vi "ESP32 BLE Client - Bluegiga.vi"() -> ()   [LabVIEW 2016]
uses:
  Typedef/BLE - State.ctl
  <vilib>/BLE/type_def/connection_status_bundle.ctl
  <vilib>/BLE/type_def/address_type.ctl
  Typedef/BLE - ADC Resolution.ctl
panel:
  in  "Exit":bool
  in  "Tab":T1(tab)
  in  "Discover":bool
  in  "USB BLE Dongle port":refnum<visa-resource-name>
  out "Dongle Status":bool
  in  "Connect dongle":bool
  out "BLED112 Dongle Info":string
  in  "MAC Address":string="24:0A:C4:04:1C:4E"
  in  "Address type":enum8{"Public", "Random"}(ring)
  in  "Connect BLE":bool
  out "BLE Status":bool
  out "Devices":i32(listbox)=-1
  in  "Min interval":u16=20 caption="Connection interval (min)" min=10 max=4000 step=1 format="%.0fms"
  in  "Max interval":u16=50 caption="Connection interval (max)" min=10 max=4000 step=1 format="%.0fms"
  in  "Latency":u16 max=500 step=1
  in  "Timeout":u16=1000 format="%.0fms"
  out "Gatt server table":i32(listbox)=-1
  in  "Single read":bool
  in  "Stream data":bool
  out "Data chart":T2(graph)
  in  "Acq interval":u32=50 min=50 max=100 step=5 format="%.0fms"
  out "Read Value":u32 caption="Read Value (Max 4 Bytes)" format="%08x"
  out "Cycle time":u32 format="%.0fms"
  in  "Clear Plot":bool
  in  "Handle":u16=42 format="%04x"
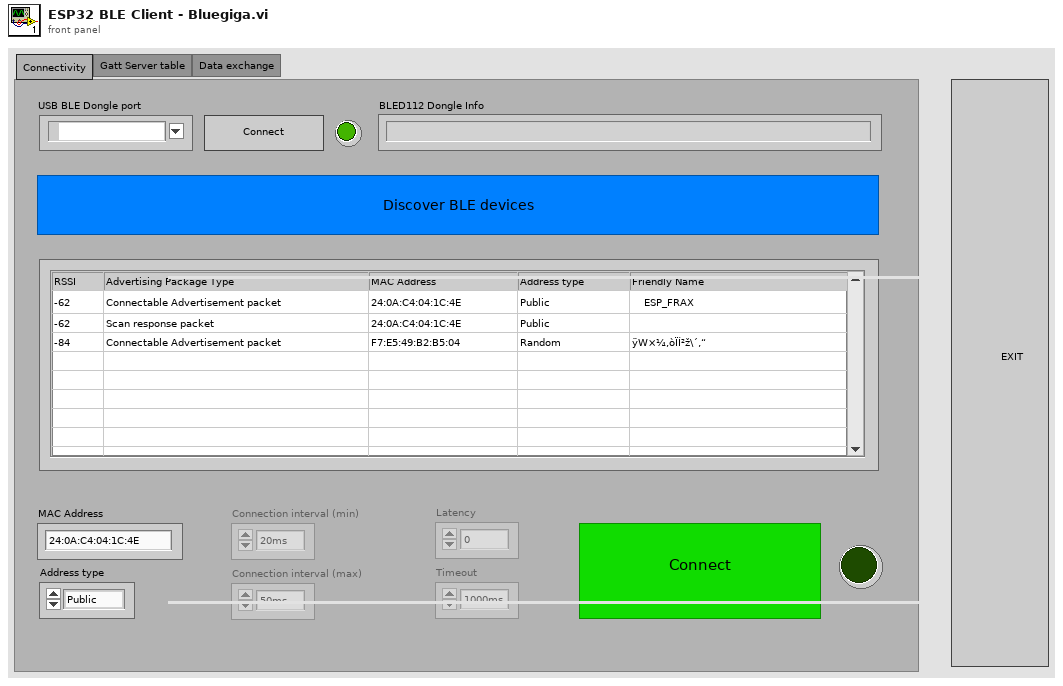
[diagram p1: front panel]
types:
  T1 = enum32{"Connectivity", "Gatt Server table", "Data exchange"}
  T2 = cluster{"Data value[0]":sgl, "Data value[1]":sgl}
  T3 = typedef "connection_status_bundle.ctl" = cluster{"MAC Address":string, "cnx handle":u8, "cnx flags":u8, "Address Type":T4, "Connection Interval (ms)":u16, "Timeout(ms)":u16, "Latency":u16, "bonding handle":u8}
  T4 = typedef "address_type.ctl" = u8
  T5 = cluster{"Connection Status":T3, "MAC Address":string, "Handle table":string[][], "Is Connected":bool}
  T6 = typedef "BLE - State.ctl" = enum16{"Connect Dongle", "Discover BLE", "Connect BLE", "Disconnect BLE", "Discover Services", "Single read", "Stream Data", "Stop Data", "Exit"}
  T7 = cluster{"Data value[0]":sgl, "Data value[1]":sgl}[]
  T8 = typedef "BLE - ADC Resolution.ctl" = enum16{"9bit", "10bit", "11bit", "12bit"}
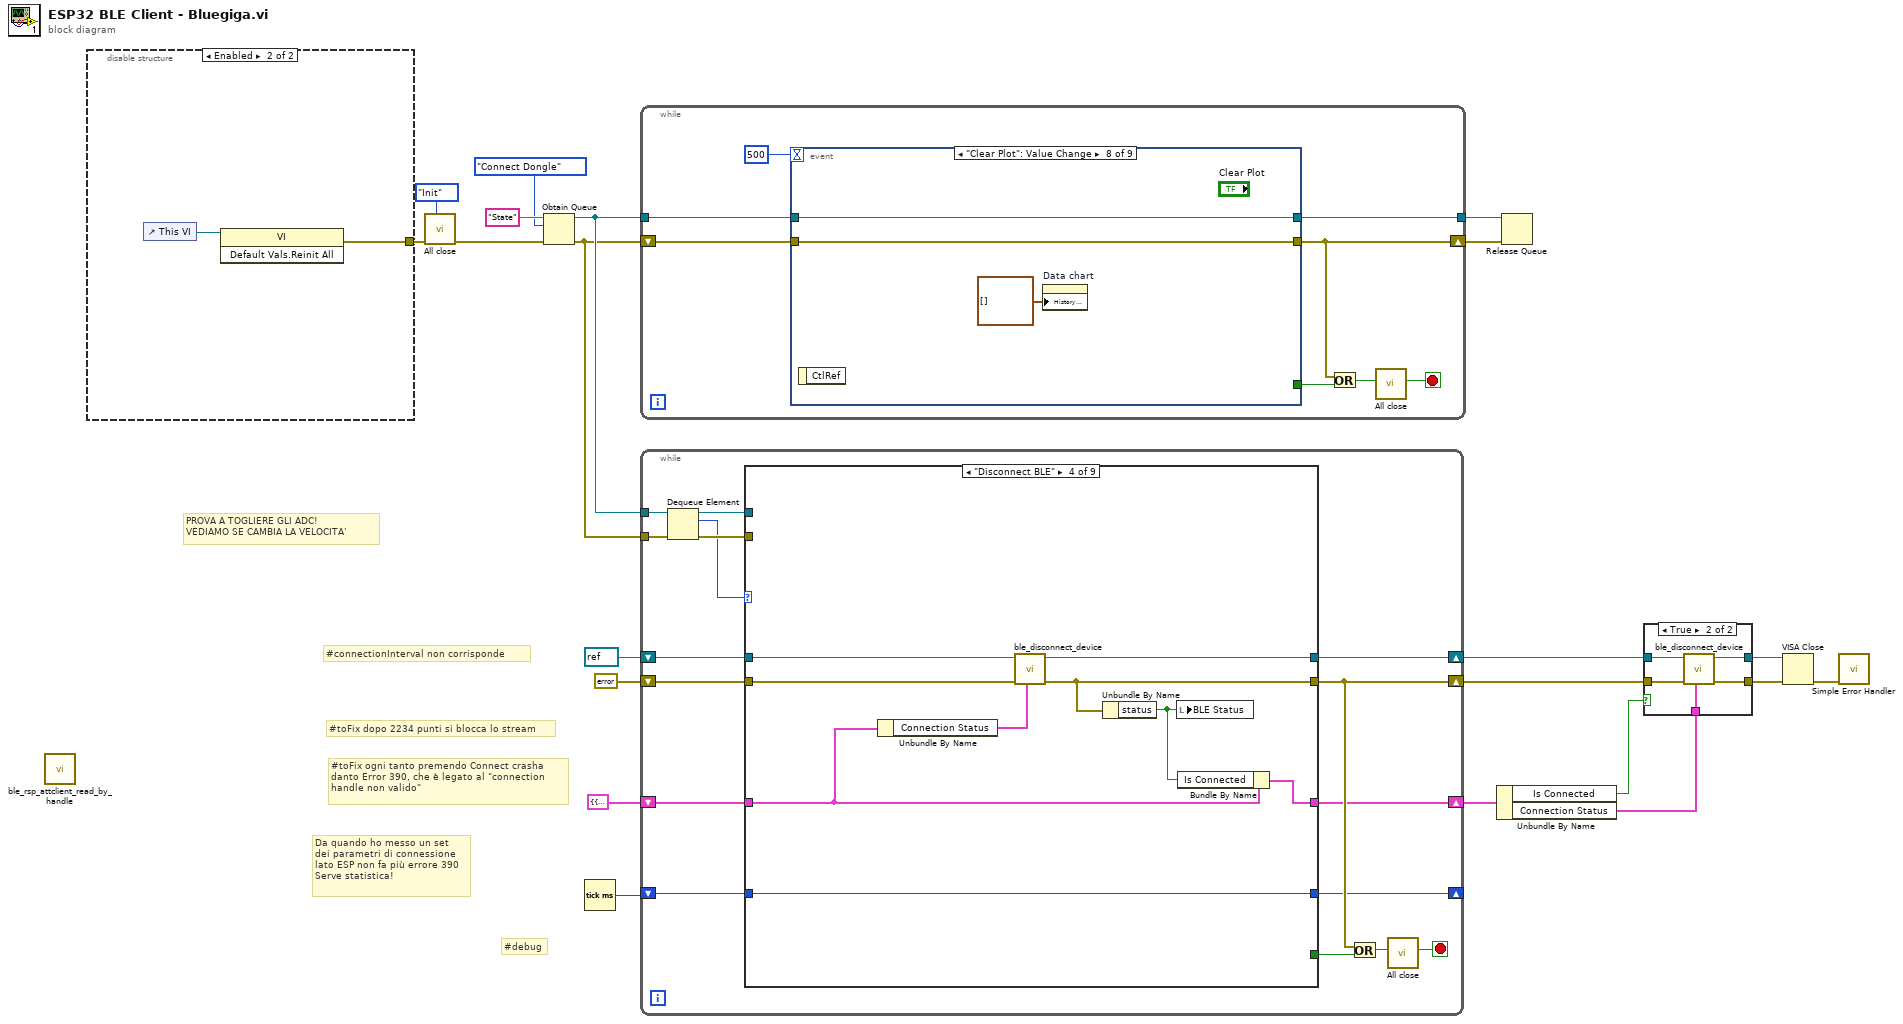
[diagram p0: block diagram]
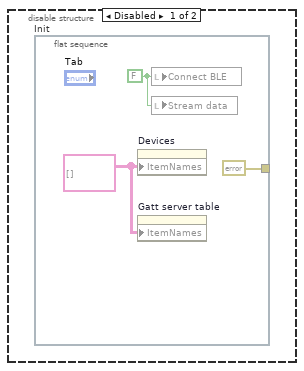
[diagram p2: hidden frame]
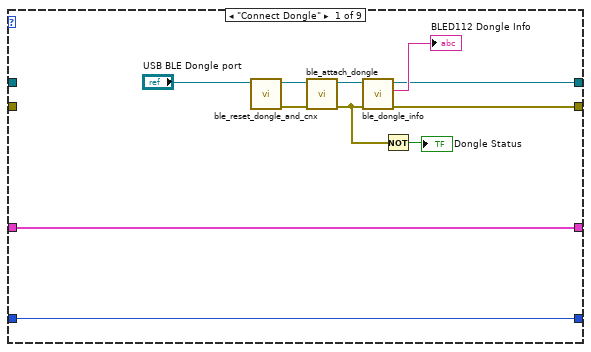
[diagram p4: hidden frame]
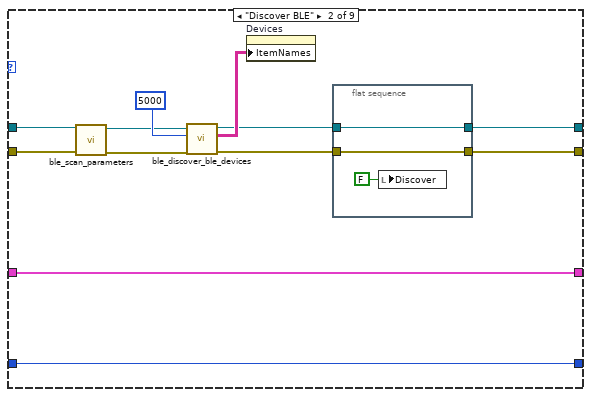
[diagram p5: hidden frame]
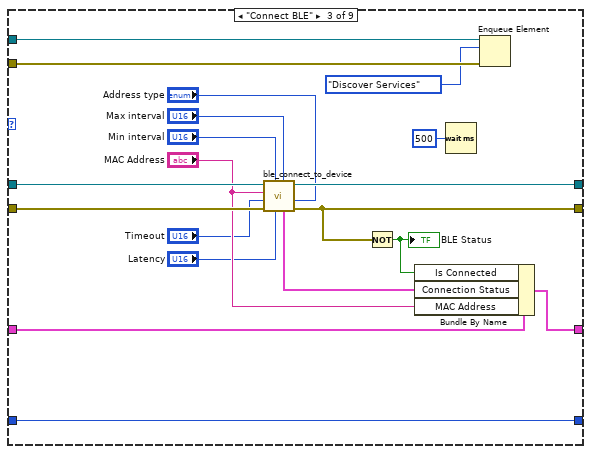
[diagram p6: hidden frame]
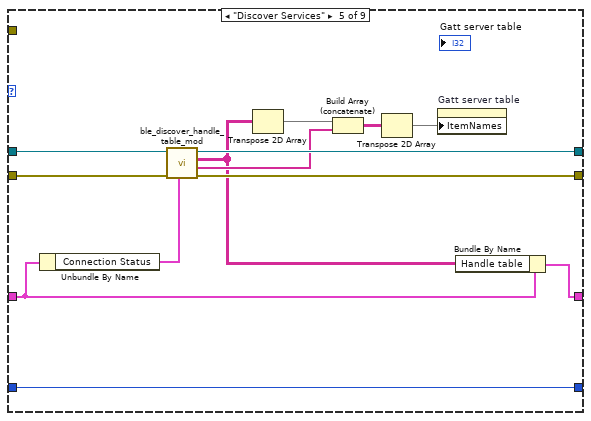
[diagram p7: hidden frame]
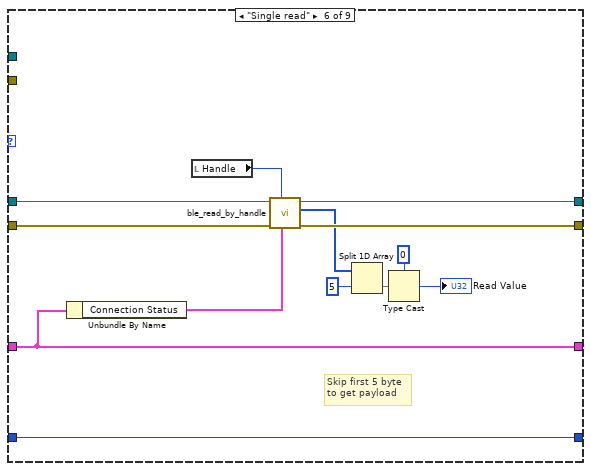
[diagram p8: hidden frame]
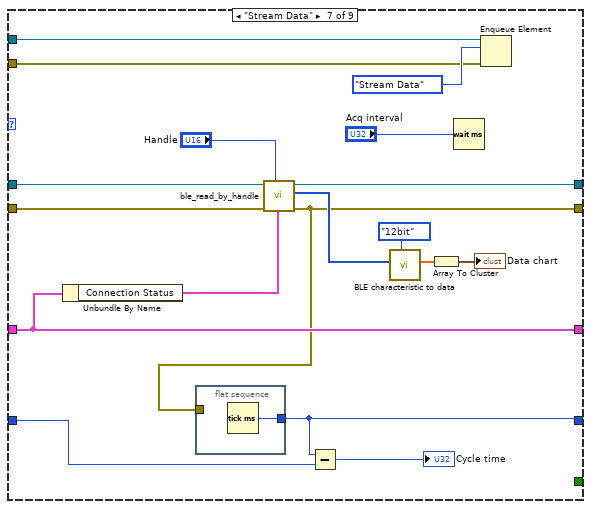
[diagram p9: hidden frame]
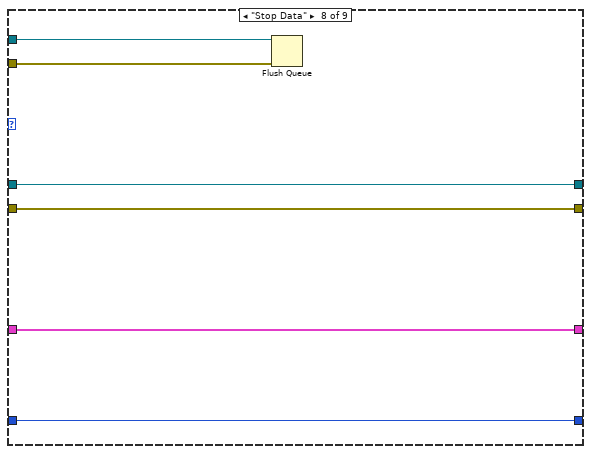
[diagram p10: hidden frame]
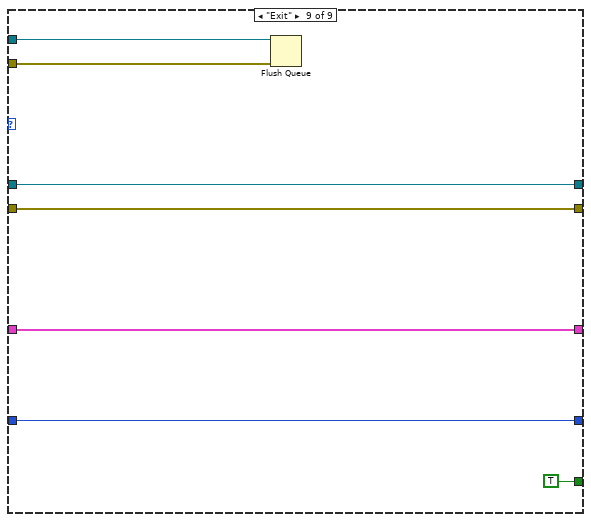
[diagram p11: hidden frame]
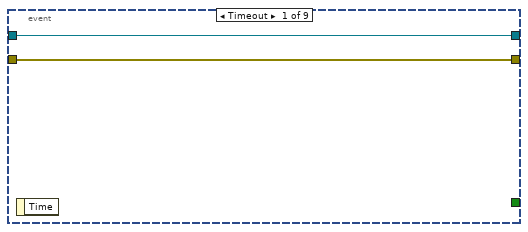
[diagram p12: hidden frame]
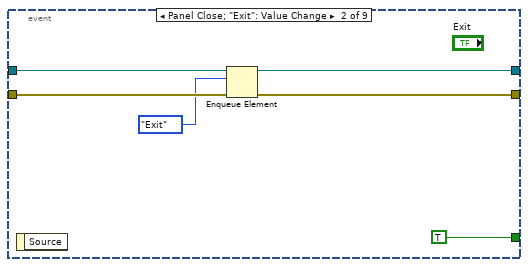
[diagram p13: hidden frame]
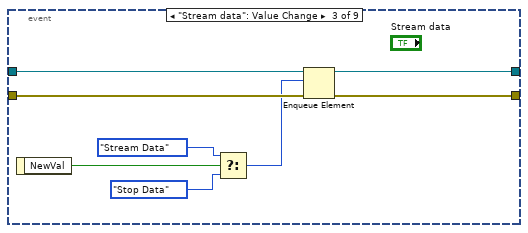
[diagram p14: hidden frame]
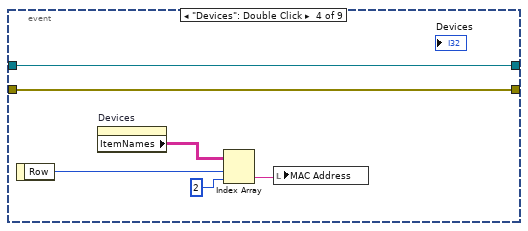
[diagram p15: hidden frame]
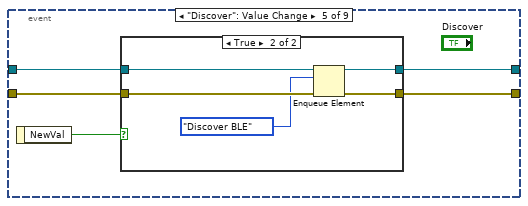
[diagram p16: hidden frame]
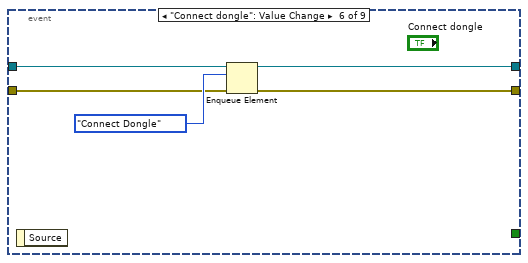
[diagram p18: hidden frame]
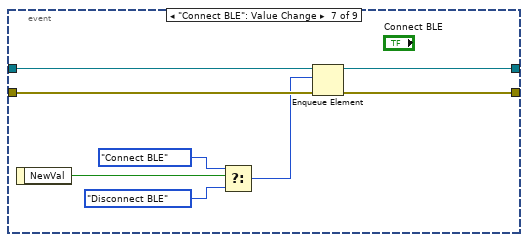
[diagram p19: hidden frame]
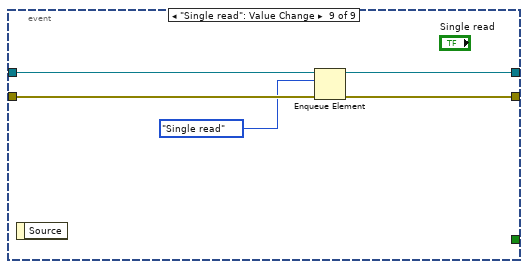
[diagram p20: hidden frame]
diagram:
  # "PROVA A TOGLIERE GLI ADC!\nVEDIAMO SE CAMBIA LA VELOCITA'"
  # "#debug"
  # "Da quando ho messo un set\ndei parametri di connessione\nlato ESP non fa più errore 390\nServe statistica!"
  # "#toFix ogni tanto premendo Connect crasha\ndanto Error 390, che è legato al \"connection\nhandle non valido\""
  # "#toFix dopo 2234 punti si blocca lo stream"
  # "#connectionInterval non corrisponde"
  n1 = call <vilib>:"ble_rsp_attclient_read_by_handle.vi"() -> ()  [unwired: 8 in, 4 out]
  n2 = disable-structure shown="Enabled" {
    disable-tunnel: [_ w25] -> w1
    frame Disabled {
      n3 = flat-sequence "Init" {
        tunnel: [errorcluster {"status"=FALSE, "code"=0, "source"=""} ("Error In")] -> _
        frame #0 {
          w22 = FALSE ("Connect BLE")
          w23 = string[][] [] ("Item Names")
          n4 = property on="Devices" class="MCListbox (strict)"("ItemNames"=w23) -> ()  [unwired: 2 in, 2 out]
          n5 = property on="Gatt server table" class="MCListbox (strict)"("ItemNames"=w23) -> ()  [unwired: 2 in, 2 out]
          n6 = local write "Connect BLE"(w22) -> ()
          n7 = local write "Stream data"(w22) -> ()
        }
      }
    }
    frame Enabled {
      n8 = control-ref of="This VI"() -> (w26:refnum<vi>)
      n9 = invoke class="VI" method="Default Vals.Reinit All"(reference=w26) -> (error out=w25:errorcluster)  [unwired: 2 in, 2 out]
    }
  }
  n10 = call "All close.vi"("Operation (Check)"=enum16{"Init", "Check"}."Init", "Error In"=w1) -> ("Error Out"=w12:errorcluster)  [unwired: 8 in, 1 out]
  n11 = Obtain Queue(name (unnamed)="State", element data type=BLE_-_State."Connect Dongle", error in (no error)=w12) -> (queue out=w18:refnum<queue>, error out=w17:errorcluster)  [unwired: 2 in, 1 out]
  n12 = Tick Count (ms)() -> (millisecond timer value=w2:u32)
  n13 = while {
    tunnel: w18 -> [w32]
    shift-right: [w29] -> w19
    shift-left: w17 -> [w33]
    tunnel: [w31] -> w20
    stop <- w27 stop-if-true
    n14 = event shown="[7] \"Clear Plot\": Value Change" {
      selector: _ -> [_ _ _ _ _ _ _ _ _]
      dyn-events: _ -> [_ _ _ _ _ _ _ _ _]
      timeout: 500 -> [_ _ _ _ _ _ _ _ _]
      tunnel: w33 -> [w35 w42 w49 w52 w60 w71 w80 w83 w88]
      tunnel: w32 -> [w36 w39 w50 w51 w61 w72 w81 w84 w89]
      tunnel: [w36 w38 w48 w51 w59 w69 w78 w84 w86] -> w31
      tunnel: [w35 w40 w47 w52 w58 w70 w79 w83 w87] -> w29
      tunnel: [_ TRUE _ _ _ _ _ _ _] -> w30
      event Timeout {
        n15 = event-data() -> ()  [unwired: 1 in, 1 out]
      }
      event Panel Close; "Exit": Value Change {
        n16 = event-data() -> ()  [unwired: 1 in, 1 out]
        n17 = Enqueue Element(queue=w39, element=BLE_-_State."Exit", error in (no error)=w42) -> (queue out=w38:refnum<queue>, error out=w40:errorcluster)  [unwired: 1 in, 1 out]
      }
      event "Stream data": Value Change {
        n18 = event-data() -> ("NewVal"=w46:bool)  [unwired: 1 in]
        n19 = Select(t=BLE_-_State."Stream Data" ("element"), s=w46, f=BLE_-_State."Stop Data") -> (s? t:f=w45:T6)
        n20 = Enqueue Element(queue=w50, element=w45, error in (no error)=w49) -> (queue out=w48:refnum<queue>, error out=w47:errorcluster)  [unwired: 1 in, 1 out]
      }
      event "Devices": Double Click {
        n21 = event-data() -> ("Row"=w55:i32)  [unwired: 1 in]
        n22 = property on="Devices" class="MCListbox (strict)"() -> ("ItemNames"=w54:string[][])  [unwired: 2 in, 2 out]
        n23 = Index Array(array=w54, index (row)=w55, index (col)=2 ("disabled index (col)")) -> (element=w53:string)
        n24 = local write "MAC Address"(w53) -> ()
      }
      event "Discover": Value Change {
        n25 = event-data() -> ("NewVal"=w57:bool)  [unwired: 1 in]
        n26 = case shown="True" w57 {
          tunnel: w61 -> [w63 w68]
          tunnel: w60 -> [w62 w67]
          tunnel: [w63 w66] -> w59
          tunnel: [w62 w65] -> w58
          frame False {
          }
          frame True {
            n27 = Enqueue Element(queue=w68, element=BLE_-_State."Discover BLE", error in (no error)=w67) -> (queue out=w66:refnum<queue>, error out=w65:errorcluster)  [unwired: 1 in, 1 out]
          }
        }
      }
      event "Connect dongle": Value Change {
        n28 = event-data() -> ()  [unwired: 1 in, 1 out]
        n29 = Enqueue Element(queue=w72, element=BLE_-_State."Connect Dongle", error in (no error)=w71) -> (queue out=w69:refnum<queue>, error out=w70:errorcluster)  [unwired: 1 in, 1 out]
      }
      event "Connect BLE": Value Change {
        n30 = event-data() -> ("NewVal"=w77:bool)  [unwired: 1 in]
        n31 = Select(t=BLE_-_State."Connect BLE", s=w77, f=BLE_-_State."Disconnect BLE" ("element")) -> (s? t:f=w74:T6)
        n32 = Enqueue Element(queue=w81, element=w74, error in (no error)=w80) -> (queue out=w78:refnum<queue>, error out=w79:errorcluster)  [unwired: 1 in, 1 out]
      }
      event "Clear Plot": Value Change {
        n33 = event-data() -> ()  [unwired: 1 in, 1 out]
        n34 = property on="Data chart" class="WFChart (strict)"("History Data"=T7 []) -> ()  [unwired: 2 in, 2 out]
      }
      event "Single read": Value Change {
        n35 = event-data() -> ()  [unwired: 1 in, 1 out]
        n36 = Enqueue Element(queue=w89, element=BLE_-_State."Single read" ("t"), error in (no error)=w88) -> (queue out=w86:refnum<queue>, error out=w87:errorcluster)  [unwired: 1 in, 1 out]
      }
    }
    n37 = Or(x=w29, y=w30) -> (x .or. y?=w28:bool)
    n38 = call "All close.vi"("Close? (F)"=w28) -> ("Close"=w27:bool)  [unwired: 9 in, 1 out]
  }
  n39 = while {
    tunnel: w18 -> [w105]
    tunnel: w17 -> [w104]
    shift-right: [w97] -> w8
    shift-left: errorcluster {"status"=FALSE, "code"=0, "source"=""} ("error out") -> [w98]
    shift-right: [w100] -> w9
    shift-left: refnum<visa-resource-name> refnum ("COM Bluegiga out") -> [w99]
    shift-right: [w94] -> w5
    shift-left: T5 {"Connection Status"={"MAC Address"="", "cnx handle"=0, "cnx flags"=0, "Address Type"=125, "Connection Interval (ms)"=125, "Timeout(ms)"=125, "Latency"=0, "bonding handle"=0}, "MAC Address"="", "Handle table"=[], "Is Connected"=FALSE} -> [w95]
    shift-right: [w90] -> _
    shift-left: w2 -> [w91]
    stop <- w92 stop-if-true
    n40 = Dequeue Element(queue=w105, error in (no error)=w104) -> (queue out=w102:refnum<queue>, element=w101:T6, error out=w103:errorcluster)  [unwired: 1 in, 1 out]
    n41 = case shown="\"Disconnect BLE\"" w101 {
      tunnel: w103 -> [_ _ w142 _ _ _ w202 w208 w212]
      tunnel: w102 -> [_ _ w143 _ _ _ w201 w209 w213]
      tunnel: [w111 w123 w148 w157 w169 w176 w190 w207 w217] -> w100
      tunnel: [w110 w124 w146 w155 w170 w177 w186 w206 w216] -> w97
      tunnel: w99 -> [_ w121 w150 w159 w168 w179 w192 w207 w217]
      tunnel: w98 -> [_ w120 w149 w158 w167 w178 w191 w206 w216]
      tunnel: [_ _ _ _ _ _ _ _ TRUE] -> w96
      tunnel: w95 -> [w112 w127 w145 w153 w172 w184 w200 w210 w214]
      tunnel: [w112 w127 w144 w152 w171 w184 w200 w210 w214] -> w94
      tunnel: w91 -> [w106 w117 w132 w154 w160 w185 w198 w205 w211]
      tunnel: [w106 w117 w132 w154 w160 w185 w195 w205 w211] -> w90
      frame "Connect Dongle" {
        n42 = call <vilib>:"ble_reset_dongle_and_cnx.vi"("COM Bluegiga in"="USB BLE Dongle port") -> ("error out"=w115:errorcluster, "COM Bluegiga out"=w108:refnum<visa-resource-name>)  [unwired: 9 in]
        n43 = call <vilib>:"ble_attach_dongle.vi"("error in (no error)"=w115, "COM Bluegiga in"=w108) -> ("error out"=w113:errorcluster, "COM Bluegiga out"=w107:refnum<visa-resource-name>)  [unwired: 8 in]
        n44 = call <vilib>:"ble_dongle_info.vi"("error in (no error)"=w113, "COM Bluegiga in"=w107) -> ("error out"=w110:errorcluster, "info"=→"BLED112 Dongle Info":string, "COM Bluegiga out"=w111:refnum<visa-resource-name>)  [unwired: 7 in]
        n45 = Not(x=w113) -> (.not. x?=→"Dongle Status":bool)
      }
      frame "Discover BLE" {
        n46 = call <vilib>:"ble_scan_parameters.vi"("error in (no error)"=w120, "COM Bluegiga in"=w121) -> ("error out"=w119:errorcluster, "COM Bluegiga out"=w118:refnum<visa-resource-name>)  [unwired: 7 in, 1 out]
        n47 = call <vilib>:"ble_discover_ble_devices.vi"("error in (no error)"=w119, "Scan Duration (10000ms)"=u32 5000, "COM Bluegiga in"=w118) -> ("error out"=w125:errorcluster, "Devices"=w126:string[][], "COM Bluegiga out"=w122:refnum<visa-resource-name>)  [unwired: 6 in]
        n48 = property on="Devices" class="MCListbox (strict)"("ItemNames"=w126) -> ()  [unwired: 2 in, 2 out]
        n49 = flat-sequence {
          tunnel: w125 -> [w130]
          tunnel: [w130] -> w124
          tunnel: [w129] -> w123
          tunnel: w122 -> [w129]
          frame #0 {
            n50 = local write "Discover"(FALSE ("Discover")) -> ()
          }
        }
      }
      frame "Connect BLE" {
        n51 = call <vilib>:"ble_connect_to_device.vi"("Address Type"="Address type", "Connection Interval Max (95ms)"="Max interval", "Latency(0)"="Latency", "Connection Interval Min (75ms)"="Min interval", "error in (no error)"=w149, "Timeout(1000ms)"="Timeout", "MAC Address"="MAC Address", "COM Bluegiga in"=w150) -> ("error out"=w146:errorcluster, "COM Bluegiga out"=w148:refnum<visa-resource-name>, "Connection Status"=w140:T3)  [unwired: 1 in]
        n52 = Not(x=w146) -> (.not. x?=w133:bool)
        "BLE Status" <- w133
        n53 = Bundle By Name(cluster=w145, "Is Connected"=w133, "Connection Status"=w140, "MAC Address"="MAC Address") -> (w144:T5)
        n54 = Wait (ms)(milliseconds to wait=u32 500) -> ()  [unwired: 1 out]
        n55 = Enqueue Element(queue=w143, element=BLE_-_State."Discover Services", error in (no error)=w142) -> ()  [unwired: 1 in, 3 out]
      }
      frame "Disconnect BLE" {
        n56 = Unbundle By Name(w153) -> ("Connection Status"=w156:T3)
        n57 = call <vilib>:"ble_disconnect_device.vi"("Connection Status"=w156, "error in (no error)"=w158, "COM Bluegiga in"=w159) -> ("error out"=w155:errorcluster, "COM Bluegiga out"=w157:refnum<visa-resource-name>)  [unwired: 7 in]
        n58 = Unbundle By Name(w155) -> ("status"=w151:bool)
        n59 = local write "BLE Status"(w151) -> ()
        n60 = Bundle By Name(cluster=w153, "Is Connected"=w151) -> (w152:T5)
      }
      frame "Discover Services" {
        n61 = Unbundle By Name(w172) -> ("Connection Status"=w161:T3)
        n62 = call "ble_discover_handle_table_mod.vi"("Connection Status"=w161, "error in (no error)"=w167, "COM Bluegiga in"=w168) -> ("error out"=w170:errorcluster, "Handle description"=w166:string[], "Handle table"=w165:string[][], "COM Bluegiga out"=w169:refnum<visa-resource-name>)  [unwired: 5 in]
        n63 = Transpose 2D Array(2D array=w165) -> (transposed array=w164:string[][])
        n64 = Build Array (concatenate)(w164, w166) -> (w163:string[][])
        n65 = Transpose 2D Array(2D array=w163) -> (transposed array=w162:string[][])
        n66 = property on="Gatt server table" class="MCListbox (strict)"("ItemNames"=w162) -> ()  [unwired: 2 in, 2 out]
        n67 = Bundle By Name(cluster=w172, "Handle table"=w165) -> (w171:T5)
      }
      frame "Single read" {
        # "Skip first 5 byte \nto get payload"
        n68 = Unbundle By Name(w184) -> ("Connection Status"=w175:T3)
        n69 = local read "Handle"() -> (w173:u16)
        n70 = call <vilib>:"ble_read_by_handle.vi"("Connection Status"=w175, "Handle"=w173, "error in (no error)"=w178, "COM Bluegiga in"=w179) -> ("error out"=w177:errorcluster, "characteristic value"=w174:u8[], "COM Bluegiga out"=w176:refnum<visa-resource-name>)  [unwired: 5 in]
        n71 = Split 1D Array(array=w174, index=5) -> (second subarray=w182:u8[])  [unwired: 1 out]
        n72 = Type Cast(type=u32 0 ("Read Value (Max 4 Bytes)"), x=w182) -> (*(type *) &x=→"Read Value":u32)
      }
      frame "Stream Data" {
        n73 = Unbundle By Name(w200) -> ("Connection Status"=w189:T3)
        n74 = flat-sequence {
          tunnel: [w204] -> w195
          tunnel: w186 -> [_]
          frame #0 {
            n75 = Tick Count (ms)() -> (millisecond timer value=w204:u32)
          }
        }
        n76 = call <vilib>:"ble_read_by_handle.vi"("Connection Status"=w189, "Handle"="Handle", "error in (no error)"=w191, "COM Bluegiga in"=w192) -> ("error out"=w186:errorcluster, "characteristic value"=w188:u8[], "COM Bluegiga out"=w190:refnum<visa-resource-name>)  [unwired: 5 in]
        n77 = Subtract(x=w195, y=w198) -> (x-y=→"Cycle time":u32)
        n78 = call "BLE characteristic to data.vi"("ADC resolution"=BLE_-_ADC_Resolution."12bit", "characteristic value"=w188) -> ("Data value"=w194:sgl[])  [unwired: 8 in, 1 out]
        n79 = Array To Cluster(array=w194) -> (cluster=→"Data chart":T2)
        n80 = Wait (ms)(milliseconds to wait="Acq interval") -> ()  [unwired: 1 out]
        n81 = Enqueue Element(queue=w201, element=BLE_-_State."Stream Data", error in (no error)=w202) -> ()  [unwired: 1 in, 3 out]
      }
      frame "Stop Data" {
        n82 = Flush Queue(queue=w209, error in (no error)=w208) -> ()  [unwired: 3 out]
      }
      frame "Exit" {
        n83 = Flush Queue(queue=w213, error in (no error)=w212) -> ()  [unwired: 3 out]
      }
    }
    n84 = Or(x=w97, y=w96) -> (x .or. y?=w93:bool)
    n85 = call "All close.vi"("Close? (F)"=w93) -> ("Close"=w92:bool)  [unwired: 9 in, 1 out]
  }
  n86 = Unbundle By Name(w5) -> ("Is Connected"=w3:bool, "Connection Status"=w4:T3)
  n87 = Release Queue(queue=w20, error in (no error)=w19) -> ()  [unwired: 1 in, 3 out]
  n88 = case shown="True" w3 {
    tunnel: w9 -> [w219 w224]
    tunnel: w8 -> [w218 w223]
    tunnel: [w219 w222] -> w7
    tunnel: [w218 w221] -> w6
    tunnel: w4 -> [_ w220]
    frame False {
    }
    frame True {
      n89 = call <vilib>:"ble_disconnect_device.vi"("Connection Status"=w220, "error in (no error)"=w223, "COM Bluegiga in"=w224) -> ("error out"=w221:errorcluster, "COM Bluegiga out"=w222:refnum<visa-resource-name>)  [unwired: 7 in]
    }
  }
  n90 = VISA Close(VISA resource name=w7, error in (no error)=w6) -> (error out=w10:errorcluster)
  n91 = call <vilib>:"Simple Error Handler.vi"("error in (no error)"=w10) -> ()  [unwired: 4 in, 5 out]
